vi "create Snake.vi"(8 "error in (no error)":errorcluster, 10 "Coordinate":T1, 11 "Snake in":refnum<class "Snake.lvclass">) -> (0 "error out":errorcluster, 3 "Snake out":refnum<class "Snake.lvclass">)   [LabVIEW 2019, in "Snake.lvclass"]
uses:
  Snake.lvclass
  Coordinate STYP.ctl
  private/Snake Component STYP.ctl
  Direction STYP.ctl
  Snake.lvclass/Snake.ctl
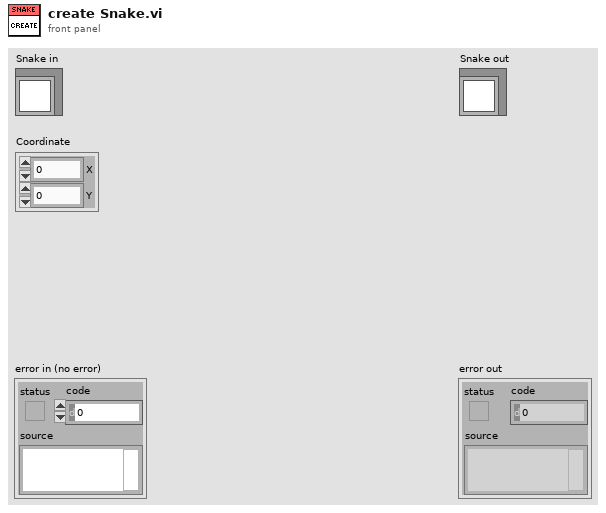
[diagram p1: front panel]
types:
  T1 = typedef "Coordinate STYP.ctl" = cluster{"X":i32, "Y":i32}
  T2 = typedef "Direction STYP.ctl" = enum16{"Up", "Down", "Left", "Right"}
  T3 = typedef "Snake.lvclass/Snake Component STYP.ctl" = cluster{"Direction":T2, "Coordinate":T1}
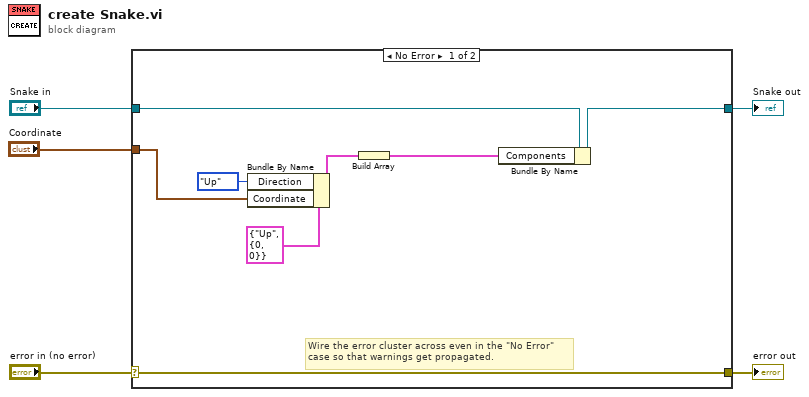
[diagram p0: block diagram]
diagram:
  n1 = case shown="No Error" "error in (no error)" {
    selector: "error in (no error)" -> [w13 w15]
    tunnel: [w13 w15] -> w4
    tunnel: [w12 w14] -> w2
    tunnel: "Snake in" -> [w11 w14]
    tunnel: "Coordinate" -> [w9 _]
    frame No Error {
      # "Wire the error cluster across even in the \"No Error\"\ncase so that warnings get propagated."
      n2 = Bundle By Name(cluster=T3 {"Direction"=enum."Up", "Coordinate"={"X"=0, "Y"=0}} ("Snake Component"), "Direction"=Direction_STYP."Up", "Coordinate"=w9) -> (w7:T3)
      n3 = Build Array(w7) -> (w6:T3[])
      n4 = Bundle By Name(cluster=w11, "Components"=w6) -> (w12:refnum<class "Snake.lvclass">)
    }
    frame Error {
    }
  }
  "error out" <- w4
  "Snake out" <- w2
